vi "Check Count.vi"(5 "source vi name":string, 6 "count power of 2":i16, 7 "buffer count":u64 format="%d elements", 8 "error in (no error)":errorcluster, 9 "offset (0)":u64 format="%d bytes", 10 "count (-1: rest)":i64=-1 format="%d elements", 11 "Pointer in":refnum<class "Pointer.lvclass">) -> (0 "error out":errorcluster, 1 "offset":u64 format="%d bytes", 2 "count":u64 format="%d elements", 3 "Pointer out":refnum<class "Pointer.lvclass">)   [LabVIEW 2020, in "Memory Manager.lvlib" / "Pointer.lvclass"]
uses:
  Pointer.lvclass
  Out of Bounds.vi
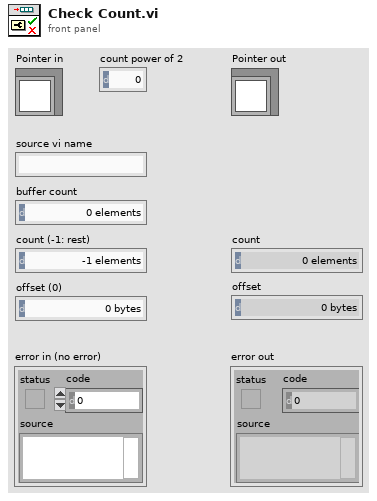
[diagram p1: front panel]
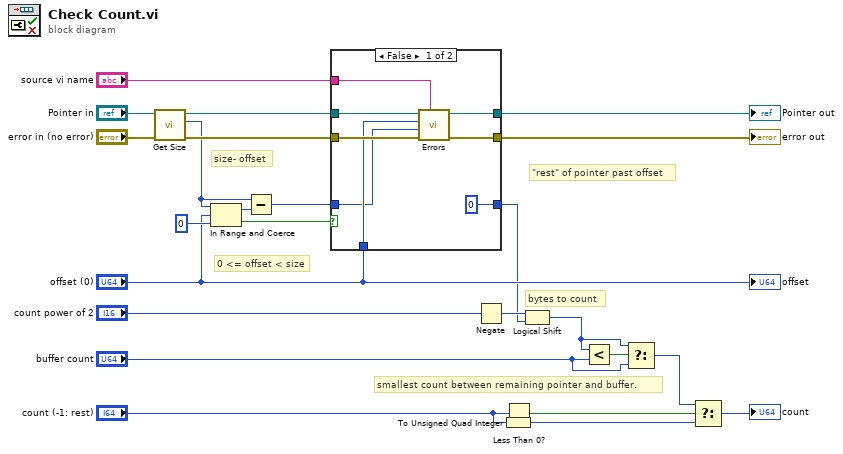
[diagram p0: block diagram]
diagram:
  # "smallest count between remaining pointer and buffer."
  # "\"rest\" of pointer past offset"
  # "bytes to count"
  # "size- offset"
  # "0 <= offset < size"
  n1 = call "Get Size.vi"("Pointer in"="Pointer in") -> ("size"=w11:u64, "Pointer out"=w18:refnum<class "Pointer.lvclass">)  [unwired: 9 in]
  n2 = In Range and Coerce(upper limit=w11, x="offset (0)", lower limit=u64 0) -> (coerced(x)=w10:u64, In Range?=w19:bool)
  n3 = Subtract(x=w11, y=w10) -> (x-y=w9:u64)
  n4 = case shown="False" w19 {
    tunnel: w18 -> [w31 w34]
    tunnel: "error in (no error)" -> [w30 w33]
    tunnel: [w29 w34] -> w16
    tunnel: [w28 w33] -> w15
    tunnel: "source vi name" -> [w27 _]
    tunnel: "offset (0)" -> [w26 _]
    tunnel: w9 -> [w25 w32]
    tunnel: [u64 0 ("t") w32] -> w7
    frame False {
      n5 = call-poly "Errors.vi"("error source vi name"=w27, "error in (no error)"=w30, "size"=w25, "offset"=w26, "Pointer in"=w31) -> ("error out"=w28:errorcluster, "Pointer out"=w29:refnum<class "Pointer.lvclass">)  [unwired: 5 in]
    }
    frame True {
    }
  }
  "error out" <- w15
  "Pointer out" <- w16
  n6 = Negate(x="count power of 2") -> (-x=w13:i16)
  n7 = To Unsigned Quad Integer(1:"count (-1: rest)") -> (0:w22:u64)
  n8 = Less Than 0?(x="count (-1: rest)") -> (x < 0?=w21:bool)
  n9 = Logical Shift(y=w13, x=w7) -> (x << y=w2:u64)
  n10 = Less?(x=w2, y="buffer count") -> (x < y?=w4:bool)
  n11 = Select(t=w2, s=w4, f="buffer count") -> (s? t:f=w1:u64)
  n12 = Select(t=w1, s=w21, f=w22) -> (s? t:f=→"count":u64)
  "offset" <- "offset (0)"
